vi "Get Metadata.vi"(8 "error in (no error)":errorcluster, 11 "ONNX Class in":refnum<class "ONNX Class.lvclass">) -> (0 "error out":errorcluster, 2 "Metadata":string[][](table), 3 "ONNX Class out":refnum<class "ONNX Class.lvclass">)   [LabVIEW 2017, in "ONNX Class Library.lvlib" / "ONNX Class.lvclass"]
uses:
  ONNX Class.lvclass
  ONNX Class Library.lvlib
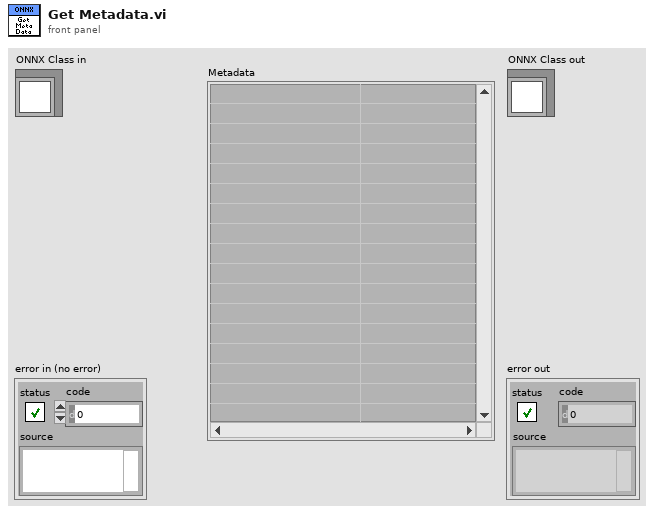
[diagram p1: front panel]
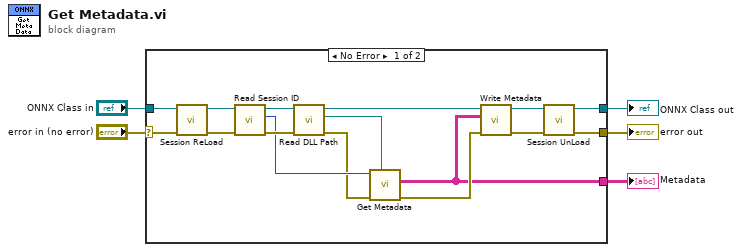
[diagram p0: block diagram]
diagram:
  n1 = case shown="No Error" "error in (no error)" {
    selector: "error in (no error)" -> [w19 w23]
    tunnel: [w7 w23] -> w4
    tunnel: [w8 w22] -> w2
    tunnel: "ONNX Class in" -> [w20 w22]
    tunnel: [w6 _] -> w1
    frame No Error {
      n2 = call-dynamic "Session ReLoad.vi"("error in (no error)"=w19, "ONNX Class in"=w20) -> ("error out"=w17:errorcluster, "ONNX Class out"=w18:refnum<class "ONNX Class.lvclass">)  [unwired: 8 in]
      n3 = call-dynamic "Read Session ID.vi"("error in (no error)"=w17, "ONNX Class in"=w18) -> ("error out"=w15:errorcluster, "Session ID"=w14:i32, "ONNX Class out"=w16:refnum<class "ONNX Class.lvclass">)  [unwired: 7 in]
      n4 = call-dynamic "Read DLL Path.vi"("error in (no error)"=w15, "ONNX Class in"=w16) -> ("error out"=w13:errorcluster, "DLL Path"=w12:path, "ONNX Class out"=w11:refnum<class "ONNX Class.lvclass">)  [unwired: 7 in]
      n5 = call "Get Metadata.vi"("DLL path"=w12, "error in (no error)"=w13, "session id in"=w14) -> ("error out"=w21:errorcluster, "Metadata"=w6:string[][])  [unwired: 6 in, 1 out]
      n6 = call-dynamic "Write Metadata.vi"("error in (no error)"=w21, "Metadata"=w6, "ONNX Class in"=w11) -> ("error out"=w9:errorcluster, "ONNX Class out"=w10:refnum<class "ONNX Class.lvclass">)  [unwired: 7 in]
      n7 = call-dynamic "Session UnLoad.vi"("error in (no error)"=w9, "ONNX Class in"=w10) -> ("error out"=w7:errorcluster, "ONNX Class out"=w8:refnum<class "ONNX Class.lvclass">)  [unwired: 8 in]
    }
    frame Error {
    }
  }
  "error out" <- w4
  "ONNX Class out" <- w2
  "Metadata" <- w1
